vi "LOAD.vi"(8 "error in (no error)":errorcluster, 9 "D(0)":dbl, 10 "Cp (1E-7 F)":dbl=1e-07, 11 "VISA resource name":refnum<visa-resource-name>) -> (0 "error out":errorcluster, 1 "LD":dbl, 2 "LC":dbl, 3 "VISA resource name out":refnum<visa-resource-name>)   [LabVIEW 2016]
panel:
  in  "Load Capacitance Threshold (1E-7 F)":dbl=1e-07
  in  "Load Supplementary Threshold (0)":dbl
  in  "Enable Load Correction (F: Disable) 2":bool
  in  "Load Correction  (0: Parallel - Dissipation Factor) 2":u16(ring) items=["Parallel - Dissipation Factor", "Parallel - Quality Factor", "Parallel - Conductance", "Parallel - Parallel Resistance", "Series - Dissipation Factor", "Series - Quality Factor", "Series- Series resistance"]
  in  "Load Correction  (0: Parallel - Dissipation Factor)":u16(ring) items=["Parallel - Dissipation Factor", "Parallel - Quality Factor", "Parallel - Conductance", "Parallel - Parallel Resistance", "Series - Dissipation Factor", "Series - Quality Factor", "Series- Series resistance"]
  in  "Enable Short Correction (F: Disable)":bool
  in  "Short Supplementary Threshold (0)":dbl
  in  "Short Capacitance Threshold (0)":dbl
  in  "Short Correction Type (0: Resistance- Reactance)":u16(ring) items=[" Resistance- Reactance", "Series Inductance- Series Resistance"]
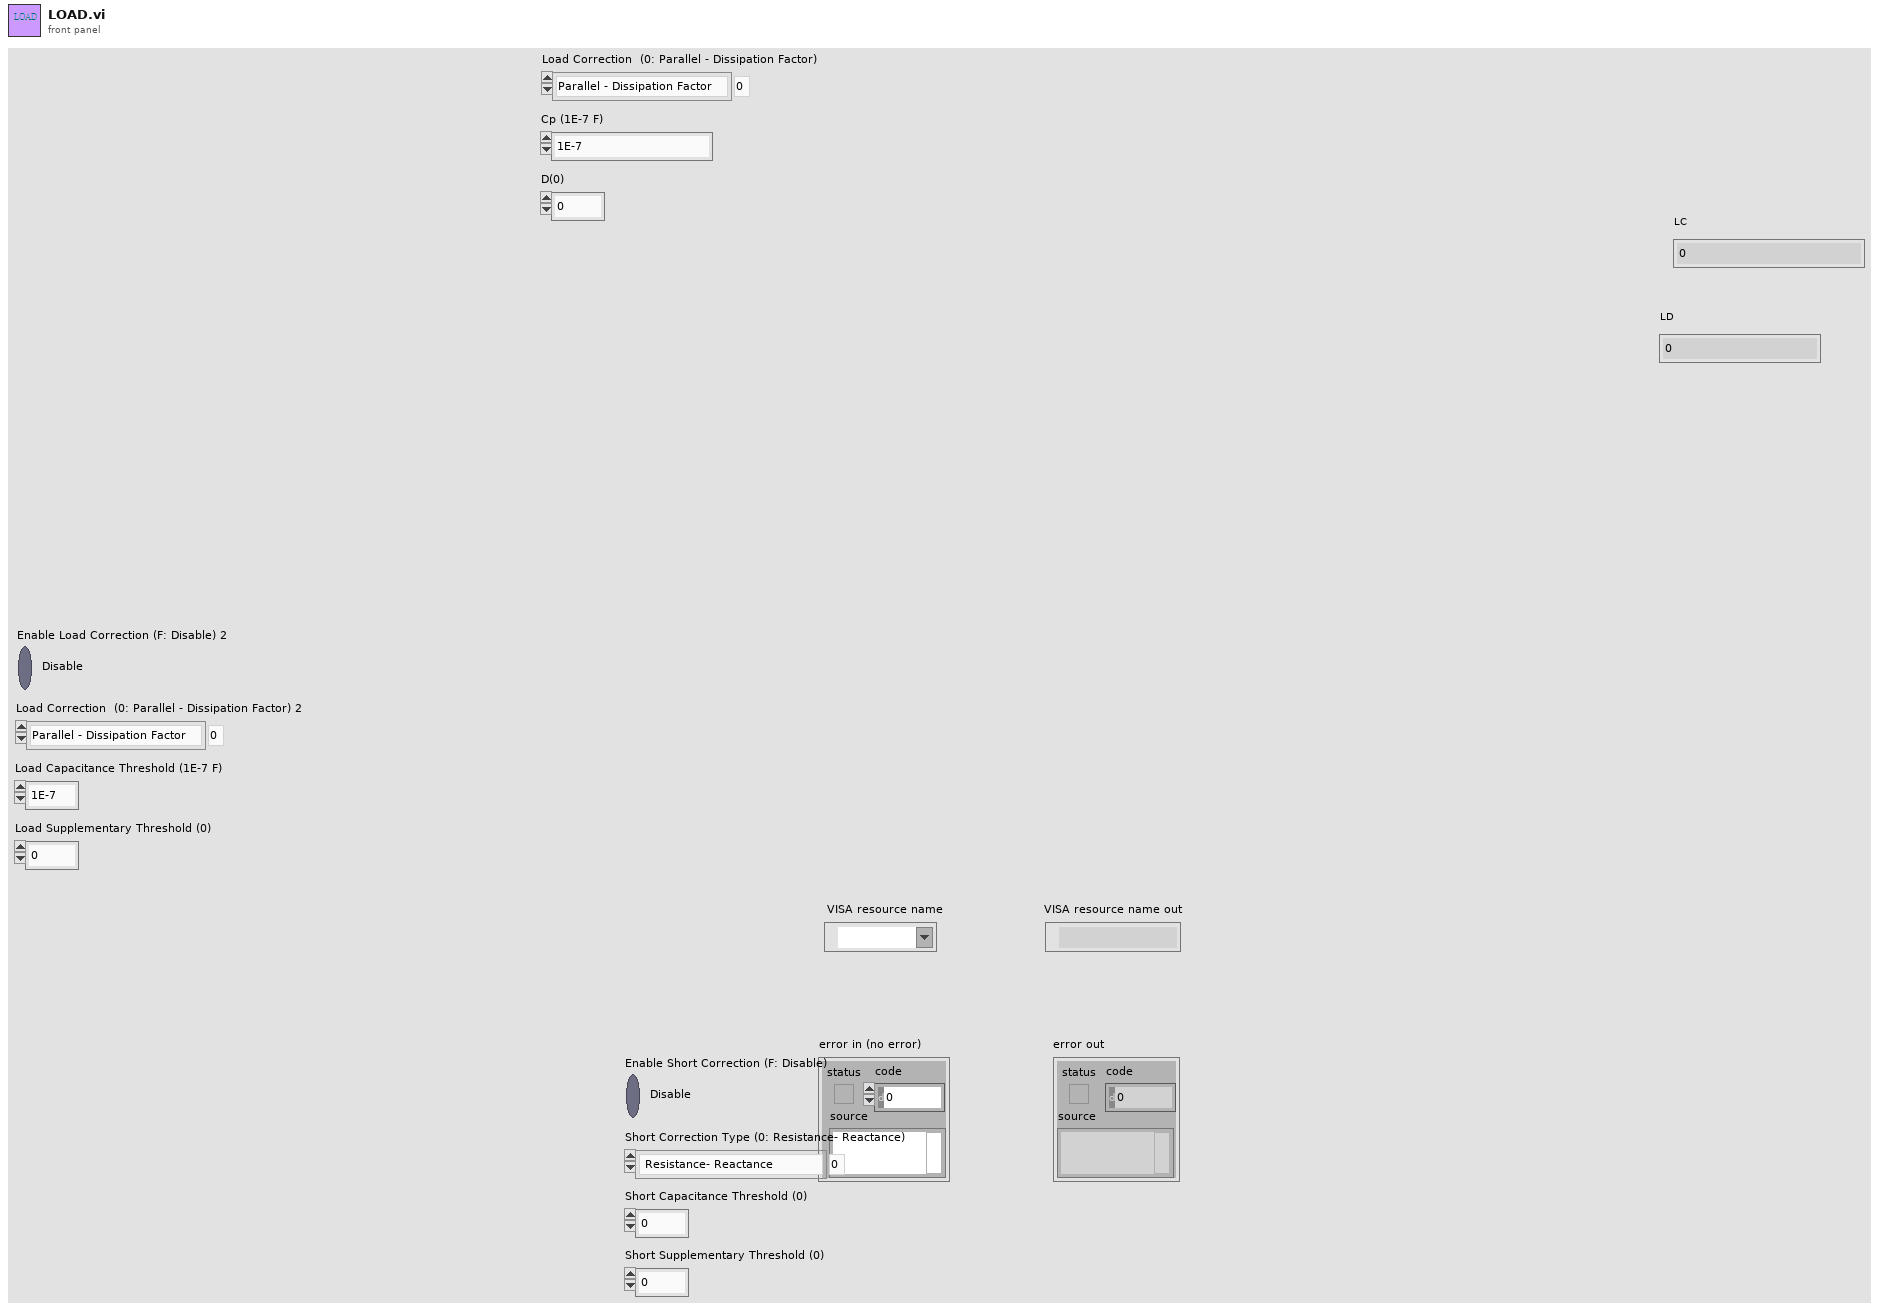
[diagram p1: front panel]
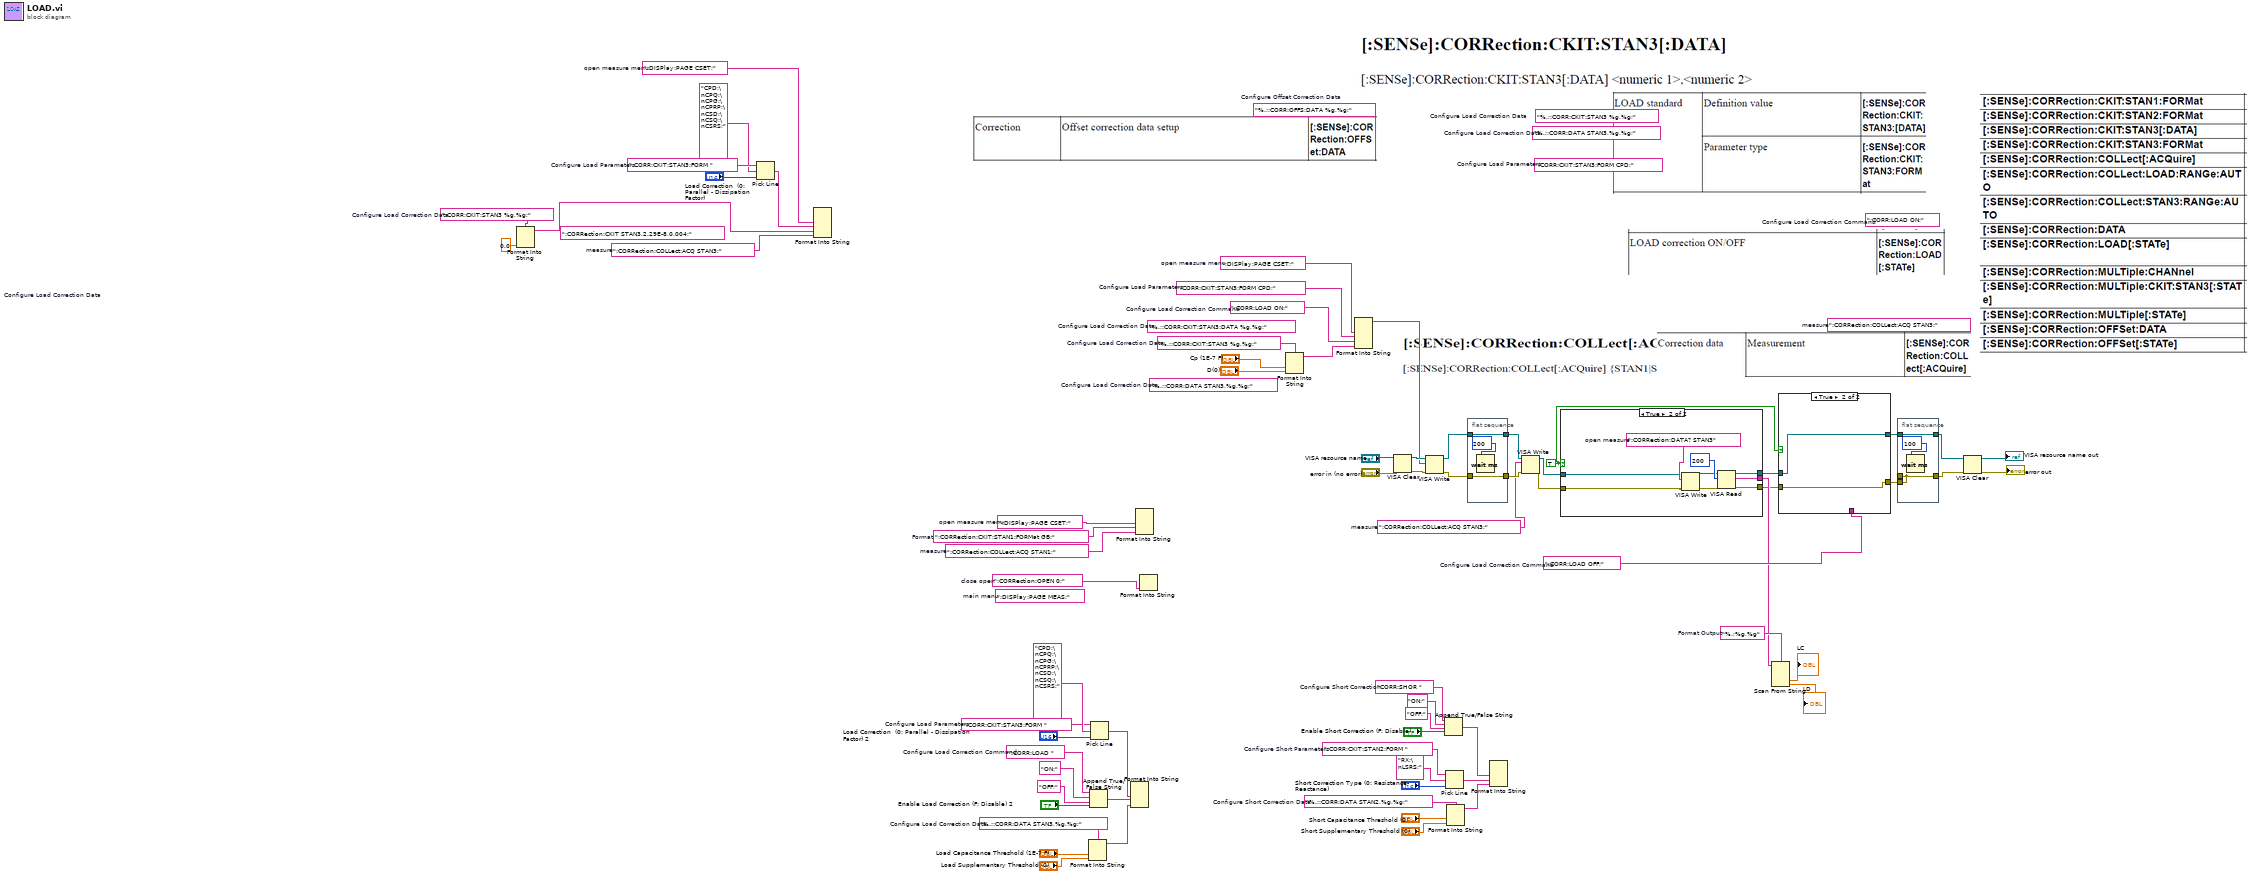
[diagram p0: block diagram]
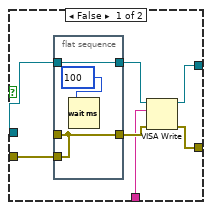
[diagram p2: hidden frame]
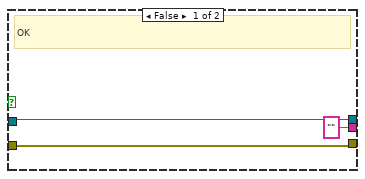
[diagram p3: hidden frame]
diagram:
  w1 = TRUE
  w7 = "%.;%g,%g"  # Format Output
  w13 = ":CORR:LOAD OFF;"  # Configure Load Correction Command
  (unwired) "%.;:CORR:DATA STAN3,%g,%g;"  # Configure Load Correction Data
  (unwired) "%.;:CORR:CKIT:STAN3:DATA %g,%g;"  # Configure Load Correction Data
  w10 = "%.;:CORR:CKIT:STAN3 %g,%g;"  # Configure Load Correction Data
  (unwired) "%.;:CORR:DATA STAN3,%g,%g;"  # Configure Load Correction Data
  w18 = ":CORRection:COLLect:ACQ STAN3;"  # measure
  (unwired) "%.;:CORR:CKIT:STAN3 %g,%g;"  # Configure Load Correction Data
  (unwired) ":CORR:LOAD ON;"  # Configure Load Correction Command
  (unwired) ":CORRection:COLLect:ACQ STAN3;"  # measure
  (unwired) ":CORR:CKIT:STAN3:FORM CPD;"  # Configure Load Parameters
  (unwired) "%.;:CORR:OFFS:DATA %g,%g;"  # Configure Offset Correction Data
  w26 = 0.0 ("input 1")
  w11 = ":CORR:LOAD ON;"  # Configure Load Correction Command
  w28 = ":DISPlay:PAGE CSET;"  # open measure menu
  w27 = ":CORR:CKIT:STAN3:FORM CPD;"  # Configure Load Parameters
  w36 = "%.;:CORR:DATA STAN3,%g,%g;"  # Configure Load Correction Data
  w34 = ":CORR:CKIT:STAN3:FORM "  # Configure Load Parameters
  w30 = ":CORR:LOAD "  # Configure Load Correction Command
  w42 = ":CORR:CKIT:STAN3 %g,%g;"  # Configure Load Correction Data
  (unwired) ":CORRection:CKIT STAN3,2.29E-8,0.004;"  # Configure Load Correction Data
  w47 = ":CORRection:OPEN 0;"  # close open
  w48 = ":CORRection:COLLect:ACQ STAN1;"  # measure
  w49 = ":CORRection:CKIT:STAN1:FORMat GB;"  # Format
  (unwired) ":DISPlay:PAGE MEAS;"  # main menu
  w50 = ":DISPlay:PAGE CSET;"  # open measure menu
  w53 = ":CORR:CKIT:STAN3:FORM "  # Configure Load Parameters
  w44 = ":CORRection:COLLect:ACQ STAN3;"  # measure
  w59 = ":DISPlay:PAGE CSET;"  # open measure menu
  w64 = "%.;:CORR:DATA STAN2,%g,%g;"  # Configure Short Correction Data
  w68 = ":CORR:CKIT:STAN2:FORM "  # Configure Short Parameters
  w72 = "CORR:SHOR "  # Configure Short Correction
  n1 = Format Into String(format string=w42, w26, w26) -> (resulting string=w43:string)  [unwired: 2 in, 1 out]
  n2 = Pick Line(string ("")=w53, multi-line string="CPD;\nCPQ;\nCPG;\nCPRP;\nCSD;\nCSQ;\nCSRS;", line index="Load Correction  (0: Parallel - Dissipation Factor)") -> (output string=w51:string)
  n3 = Format Into String(w59, w51, w43, w44) -> ()  [unwired: 3 in, 2 out]
  n4 = Format Into String(format string=w36, "Load Capacitance Threshold (1E-7 F)", "Load Supplementary Threshold (0)") -> (resulting string=w40:string)  [unwired: 2 in, 1 out]
  n5 = Append True/False String(1:"Enable Load Correction (F: Disable) 2", 2:"OFF;" ("false string"), 3:"ON;" ("true string"), 4:w30) -> (0:w39:string)
  n6 = Pick Line(string ("")=w34, multi-line string="CPD;\nCPQ;\nCPG;\nCPRP;\nCSD;\nCSQ;\nCSRS;", line index="Load Correction  (0: Parallel - Dissipation Factor) 2") -> (output string=w41:string)
  n7 = Format Into String(w41, w39, w40) -> ()  [unwired: 3 in, 2 out]
  n8 = Format Into String(w50, w49, w48) -> ()  [unwired: 3 in, 2 out]
  n9 = Format Into String(w47) -> ()  [unwired: 3 in, 2 out]
  n10 = Format Into String(format string=w10, "Cp (1E-7 F)", "D(0)") -> (resulting string=w12:string)  [unwired: 2 in, 1 out]
  n11 = Format Into String(w28, w27, w11, w12) -> (resulting string=w23:string)  [unwired: 3 in, 1 out]
  n12 = VISA Clear(VISA resource name="VISA resource name", error in (no error)="error in (no error)") -> (VISA resource name out=w58:refnum<visa-resource-name>, error out=w57:errorcluster)
  n13 = VISA Write(VISA resource name=w58, write buffer=w23, error in (no error)=w57) -> (VISA resource name out=w21:refnum<visa-resource-name>, error out=w20:errorcluster)  [unwired: 1 out]
  n14 = Append True/False String(1:"Enable Short Correction (F: Disable)", 2:"OFF;" ("true string"), 3:"ON;" ("true string"), 4:w72) -> (0:w61:string)
  n15 = Pick Line(string ("")=w68, multi-line string="RX;\nLSRS;", line index="Short Correction Type (0: Resistance- Reactance)") -> (output string=w62:string)
  n16 = Format Into String(format string=w64, "Short Capacitance Threshold (0)", "Short Supplementary Threshold (0)") -> (resulting string=w60:string)  [unwired: 2 in, 1 out]
  n17 = flat-sequence {
    tunnel: [w74] -> w22
    tunnel: w21 -> [w74]
    tunnel: w20 -> [w73]
    tunnel: [w73] -> w19
    frame #0 {
      n18 = Wait (ms)(milliseconds to wait=u32 200 ("byte count")) -> ()  [unwired: 1 out]
    }
  }
  n19 = Format Into String(w61, w62, w60) -> ()  [unwired: 3 in, 2 out]
  n20 = VISA Write(VISA resource name=w22, write buffer=w18, error in (no error)=w19) -> (VISA resource name out=w4:refnum<visa-resource-name>, error out=w3:errorcluster)  [unwired: 1 out]
  n21 = case shown="True" w1 {
    tunnel: ["" ("read buffer") w83] -> w6
    tunnel: [w78 w82] -> w5
    tunnel: w4 -> [w78 w81]
    tunnel: w3 -> [w77 w80]
    tunnel: [w77 w79] -> w2
    frame False {
      # "OK"
    }
    frame True {
      w87 = ":CORRection:DATA? STAN3"  # open measure
      n22 = VISA Write(VISA resource name=w81, write buffer=w87, error in (no error)=w80) -> (VISA resource name out=w84:refnum<visa-resource-name>, error out=w85:errorcluster)  [unwired: 1 out]
      n23 = VISA Read(VISA resource name=w84, byte count=u32 200, error in (no error)=w85) -> (VISA resource name out=w82:refnum<visa-resource-name>, read buffer=w83:string, error out=w79:errorcluster)  [unwired: 1 out]
    }
  }
  n24 = Scan From String(format string=w7, input string=w6) -> (output 1=→"LC":dbl, output 2=→"LD":dbl)  [unwired: 4 in, 3 out]
  n25 = case shown="True" w1 {
    tunnel: [w92 w99] -> w17
    tunnel: [w91 w98] -> w15
    tunnel: w13 -> [w90 _]
    tunnel: w5 -> [w89 w99]
    tunnel: w2 -> [w88 w98]
    frame False {
      n26 = flat-sequence {
        tunnel: [w96] -> w93
        tunnel: w89 -> [w96]
        tunnel: [w95] -> _
        tunnel: [w95] -> w94
        tunnel: w88 -> [w95]
        frame #0 {
          n27 = Wait (ms)(milliseconds to wait=u32 100 ("byte count")) -> ()  [unwired: 1 out]
        }
      }
      n28 = VISA Write(VISA resource name=w93, write buffer=w90, error in (no error)=w94) -> (VISA resource name out=w92:refnum<visa-resource-name>, error out=w91:errorcluster)  [unwired: 1 out]
    }
    frame True {
    }
  }
  n29 = flat-sequence {
    tunnel: [w101] -> w16
    tunnel: w17 -> [w101]
    tunnel: [w100] -> _
    tunnel: [w100] -> w14
    tunnel: w15 -> [w100]
    frame #0 {
      n30 = Wait (ms)(milliseconds to wait=u32 100 ("byte count")) -> ()  [unwired: 1 out]
    }
  }
  n31 = VISA Clear(VISA resource name=w16, error in (no error)=w14) -> (VISA resource name out=→"VISA resource name out":refnum<visa-resource-name>, error out=→"error out":errorcluster)
